vi "Delete Wire.vi"(0 "Terminal Reference":refnum<vi>, 11 "error in (no error)":errorcluster) -> (15 "error out":errorcluster)   [LabVIEW 2021, in "Converter.lvlib"]
uses:
  Converter.lvlib
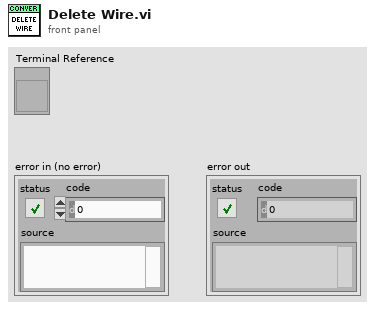
[diagram p1: front panel]
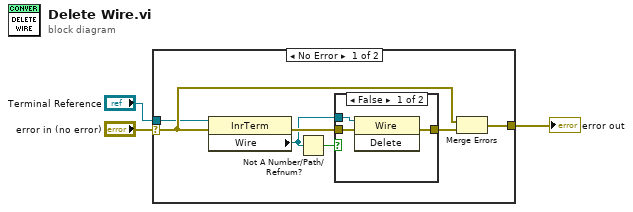
[diagram p0: block diagram]
diagram:
  n1 = case shown="No Error" "error in (no error)" {
    selector: "error in (no error)" -> [w9 w15]
    tunnel: [w10 w15] -> w3
    tunnel: "Terminal Reference" -> [w4 _]
    frame No Error {
      n2 = property class="InrTerm"(reference=w4, error in=w9) -> (error out=w7:errorcluster, "Wire"=w6:refnum<vi>)  [unwired: 1 out]
      n3 = Not A Number/Path/Refnum?(number/path/refnum=w6) -> (NaN/Path/Refnum?=w5:bool)
      n4 = case shown="False" w5 {
        tunnel: w6 -> [w13 _]
        tunnel: w7 -> [w12 w14]
        tunnel: [w11 w14] -> w8
        frame False {
          n5 = invoke class="Wire" method="Delete"(reference=w13, error in=w12) -> (error out=w11:errorcluster)  [unwired: 1 in, 2 out]
        }
        frame True {
        }
      }
      n6 = Merge Errors(w9, w8) -> (w10:errorcluster)
    }
    frame Error {
    }
  }
  "error out" <- w3
